vi "Load from DOM XML.vi"(8 "Error In":errorcluster, 10 "DOM In":refnum<k20>, 11 "UIM In":refnum<data-value>) -> (0 "Error Out":errorcluster, 2 "DOM Out":refnum<k20>, 3 "UIM Out":refnum<data-value>)   [LabVIEW 2020, in "UIM.lvlib" / "UIM.lvclass"]
doc: "Overwrite the existing UIM state data with the data loaded from XML."
uses:
  UIM.lvclass
  UIM.lvclass/UIM.ctl
  <vilib>/xml/Close Reference(Node).vi
  <resource>/objmgr/DOMUserDefRef.rc
  <vilib>/xml/NI_XML.lvlib
  UIP Interface/UIP Interface.lvclass
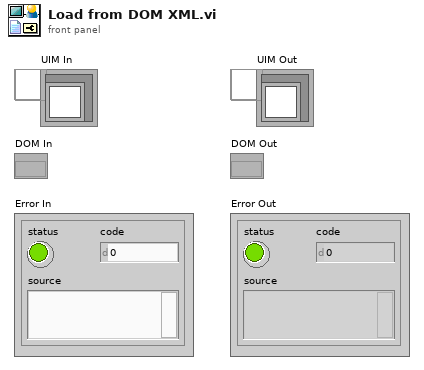
[diagram p1: front panel]
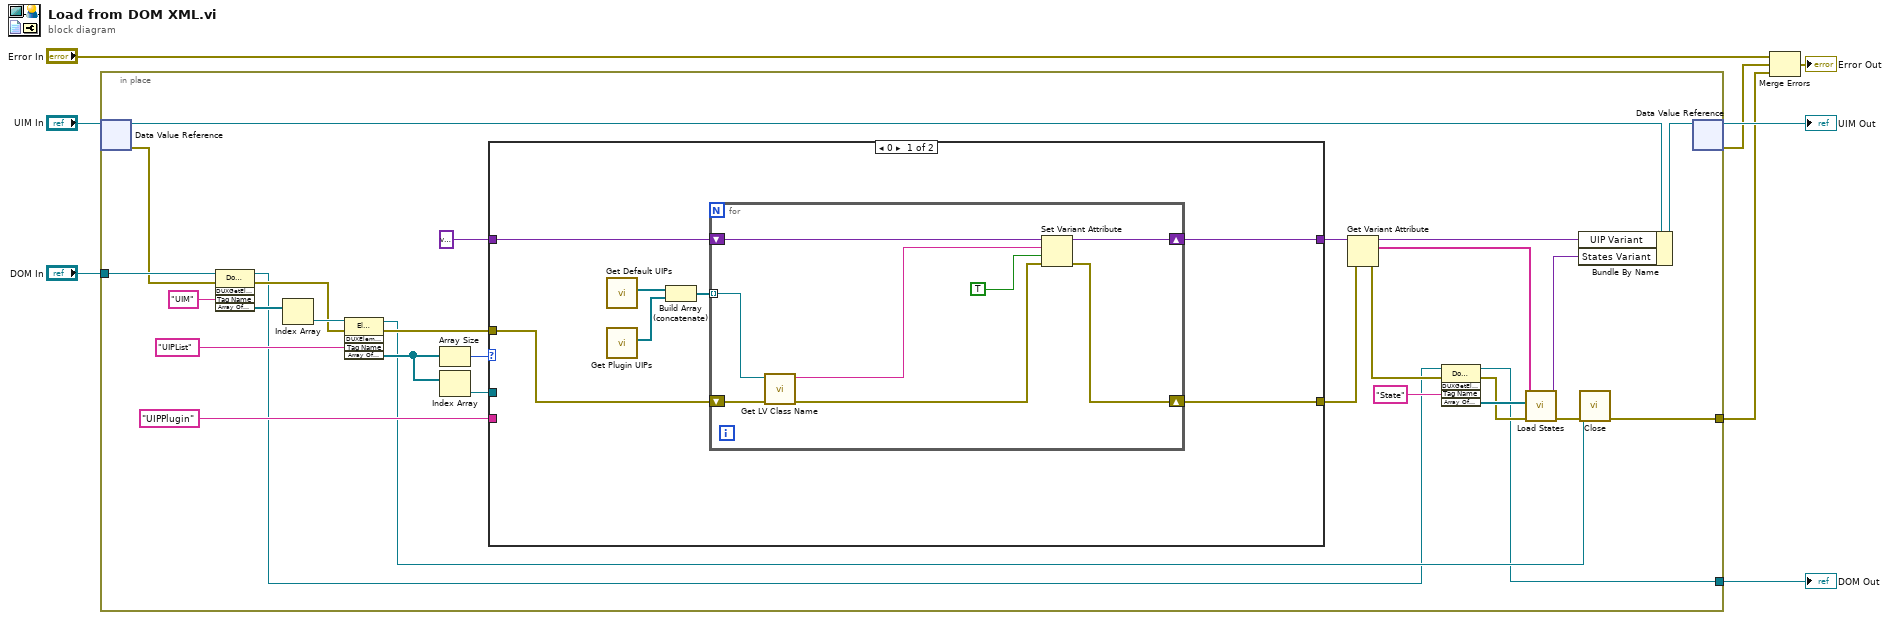
[diagram p0: block diagram]
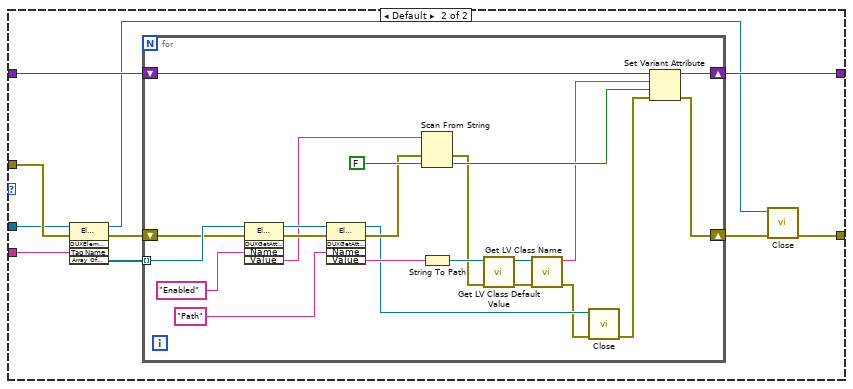
[diagram p2: hidden frame]
diagram:
  n1 = in-place {
    in-place-border: [w10] -> w4
    in-place-border: "DOM In" -> [w17]
    in-place-border: [w9] -> w1
    n2 = in-place-dvr #1("UIM In") -> (w35:refnum<class "UIM.lvclass">, w16:errorcluster)
    n3 = invoke class="Document" method="DUXGetElementsByTagName"(reference=w17, error in=w16, "Tag Name"="UIM") -> (reference out=w11:refnum<k20>, error out=w23:errorcluster, "Array Of Elements"=w30:refnum<k20>[])  [unwired: 2 in, 2 out]
    n4 = Index Array(array=w30) -> (element=w25:refnum<k20>)  [unwired: 1 in]
    n5 = invoke class="Element" method="DUXElementGetElementsByTagNameArray"(reference=w25, error in=w23, "Tag Name"="UIPList") -> (reference out=w12:refnum<k20>, error out=w18:errorcluster, "Array Of Elements"=w24:refnum<k20>[])  [unwired: 2 in, 2 out]
    n6 = Array Size(array=w24) -> (size(s)=w20:i32)
    n7 = Index Array(array=w24) -> (element=w22:refnum<k20>)  [unwired: 1 in]
    n8 = case shown="0" w20 {
      tunnel: variant -> [w42 w62]
      tunnel: [w40 w61] -> w26
      tunnel: w18 -> [w39 w58]
      tunnel: w22 -> [_ w57]
      tunnel: "UIPPlugin" ("Tag Name") -> [_ w56]
      tunnel: [w38 w54] -> w19
      frame 0 {
        n9 = call "Get Default UIPs.vi"() -> ("UIPs"=w44:refnum<class "UIP Interface.lvclass">[])  [unwired: 11 in]
        n10 = call "Get Plugin UIPs.vi"() -> ("UIPs"=w43:refnum<class "UIP Interface.lvclass">[])  [unwired: 11 in]
        n11 = Build Array (concatenate)(w44, w43) -> (w41:refnum<class "UIP Interface.lvclass">[])
        n12 = for {
          shift-right: [w47] -> w40
          shift-left: w42 -> [w52]
          tunnel: w41 -> [w50] mode=indexing
          shift-right: [w46] -> w38
          shift-left: w39 -> [w49]
          n13 = call <vilib>:"Get LV Class Name.vi"("error in (no error)"=w49, "object"=w50) -> ("error out"=w48:errorcluster, "class name"=w45:string)  [unwired: 8 in]
          n14 = Set Variant Attribute(Variant=w52, name=w45, value=TRUE, error in=w48) -> (Variant out=w47:variant, error out=w46:errorcluster)  [unwired: 1 out]
        }
      }
      frame Default {
        n15 = invoke class="Element" method="DUXElementGetElementsByTagNameArray"(reference=w57, error in=w58, "Tag Name"=w56) -> (reference out=w53:refnum<k20>, error out=w60:errorcluster, "Array Of Elements"=w59:refnum<k20>[])  [unwired: 2 in, 2 out]
        n16 = for {
          tunnel: w59 -> [w83] mode=indexing
          shift-right: [w73] -> w55
          shift-left: w60 -> [w82]
          shift-right: [w74] -> w61
          shift-left: w62 -> [w75]
          n17 = invoke class="Element" method="DUXGetAttribute"(reference=w83, error in=w82, "Name"="Enabled") -> (reference out=w81:refnum<k20>, error out=w79:errorcluster, "Value"=w78:string)  [unwired: 2 in, 2 out]
          n18 = invoke class="Element" method="DUXGetAttribute"(reference=w81, error in=w79, "Name"="Path") -> (reference out=w65:refnum<k20>, error out=w76:errorcluster, "Value"=w71:string)  [unwired: 2 in, 2 out]
          n19 = Scan From String(input string=w78, error in=w76, default 1=FALSE) -> (error out=w67:errorcluster, output 1=w72:bool)  [unwired: 2 in, 2 out]
          n20 = String To Path(string=w71) -> (path=w70:path)
          n21 = call <vilib>:"Get LV Class Default Value.vi"("error in (no error)"=w67, "class path"=w70) -> ("error out"=w69:errorcluster, "object"=w68:refnum<class>)  [unwired: 8 in]
          n22 = call <vilib>:"Get LV Class Name.vi"("error in (no error)"=w69, "object"=w68) -> ("error out"=w64:errorcluster, "class name"=w66:string)  [unwired: 8 in]
          n23 = call-poly <vilib>:"Close.vi"("error in (no error)"=w64, "node"=w65) -> ("error out"=w63:errorcluster)  [unwired: 7 in]
          n24 = Set Variant Attribute(Variant=w75, name=w66, value=w72, error in=w63) -> (Variant out=w74:variant, error out=w73:errorcluster)  [unwired: 1 out]
        }
        n25 = call-poly <vilib>:"Close.vi"("error in (no error)"=w55, "node"=w53) -> ("error out"=w54:errorcluster)  [unwired: 7 in]
      }
    }
    n26 = Get Variant Attribute(Variant=w26, error in=w19) -> (duplicate Variant=w15:variant, names=w14:string[], error out=w13:errorcluster)  [unwired: 2 in, 1 out]
    n27 = invoke class="Document" method="DUXGetElementsByTagName"(reference=w11, error in=w13, "Tag Name"="State") -> (reference out=w9:refnum<k20>, error out=w32:errorcluster, "Array Of Elements"=w36:refnum<k20>[])  [unwired: 2 in, 2 out]
    n28 = call "Load States.vi"("Error In"=w32, "States Nodes"=w36, "UIPs"=w14) -> ("Error Out"=w31:errorcluster, "States Variant"=w33:variant)  [unwired: 7 in]
    n29 = Bundle By Name(cluster=w35, "UIP Variant"=w15, "States Variant"=w33) -> (w34:refnum<class "UIM.lvclass">)
    n30 = call-poly <vilib>:"Close.vi"("error in (no error)"=w31, "node"=w12) -> ("error out"=w10:errorcluster)  [unwired: 7 in]
    n31 = in-place-dvr #1(w34) -> (→"UIM Out":refnum<data-value>, w3:errorcluster)
  }
  "DOM Out" <- w1
  n32 = Merge Errors("Error In", w3, w4) -> (→"Error Out":errorcluster)
